vi "Game controller input.vi"(0 "device ID in":refnum<k1>, 3 "error in (no error)":errorcluster) -> (5 "device ID out":refnum<k1>, 6 "Common":dbl, 7 "Diff":dbl, 8 "error out":errorcluster)   [LabVIEW 2011]
uses:
  <vilib>/Utility/inputDevices.llb/joystickAcquire.vi
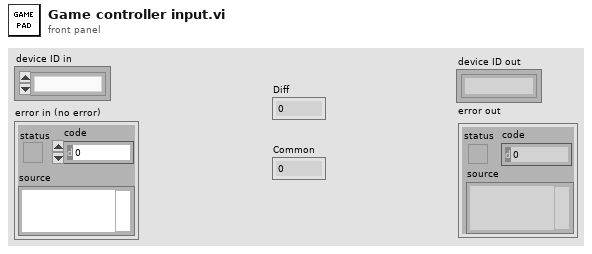
[diagram p1: front panel]
types:
  T1 = cluster{"X axis":i32, "Y axis":i32, "Z axis":i32, "X axis rotation":i32, "Y axis rotation":i32, "Z axis rotation":i32, "U axis":i32, "V axis":i32}
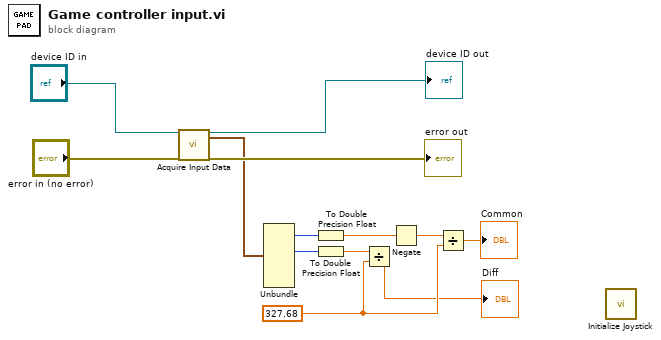
[diagram p0: block diagram]
diagram:
  w3 = 327.68
  n1 = call-poly <vilib>:"Acquire Input Data.vi"("device ID"="device ID in", "error in (no error)"="error in (no error)") -> ("device ID"=→"device ID out":refnum<k1>, "axis info"=w9:T1, "error out"=→"error out":errorcluster)  [unwired: 13 in, 2 out]
  n2 = Unbundle(w9) -> ("Y axis"=w8:i32, "X axis rotation"=w7:i32)  [unwired: 6 out]
  n3 = To Double Precision Float(number=w8) -> (double precision float=w6:dbl)
  n4 = To Double Precision Float(number=w7) -> (double precision float=w4:dbl)
  n5 = Divide(x=w4, y=w3) -> (x/y=→"Diff":dbl)
  n6 = Negate(x=w6) -> (-x=w5:dbl)
  n7 = Divide(x=w5, y=w3) -> (x/y=→"Common":dbl)
  n8 = call <vilib>:"Initialize Joystick.vi"() -> ()  [unwired: 10 in, 2 out]
